vi "setSpeedByEnum.vi"(6 "Delay between send and receive [ms]":i32=1000, 8 "error in (no error)":errorcluster, 11 "CCD in":refnum<class "CCD.lvclass">) -> (0 "error out":errorcluster, 1 "ID":i32, 2 "results-JSON string":string, 3 "CCD out":refnum<class "CCD.lvclass">)   [LabVIEW 2023, in "CCD.lvclass"]
uses:
  CCD.lvclass
  CCD.lvclass/CCD.ctl
  SpeedTokenExampleEnum.ctl
panel:
  in  "speed":T1
  # "Connector Pane"
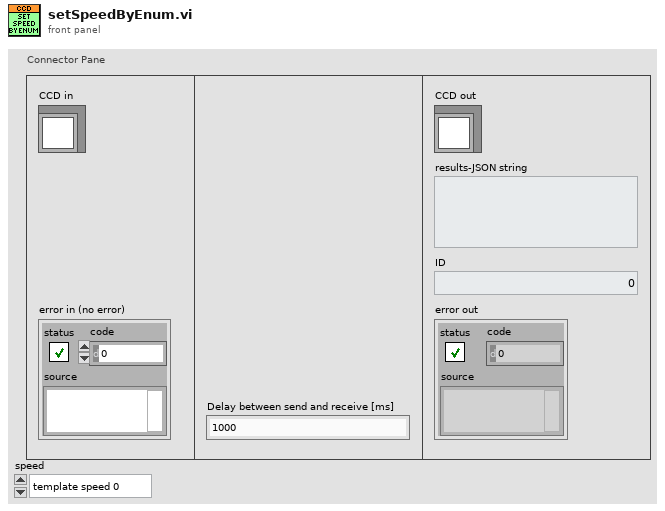
[diagram p1: front panel]
types:
  T1 = typedef "CCD.lvclass/SpeedTokenExampleEnum.ctl" = enum16{"template speed 0", "template speed 1", "template speed 2"}
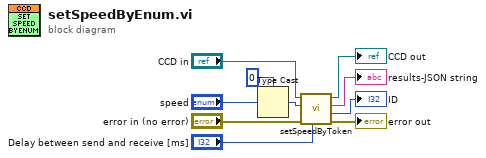
[diagram p0: block diagram]
diagram:
  n1 = Type Cast(type=u16 0, x="speed") -> (*(type *) &x=w2:u16)
  n2 = call "setSpeedByToken.vi"("Delay between send and receive [ms]"="Delay between send and receive [ms]", "error in (no error)"="error in (no error)", "speed token"=w2, "CCD in"="CCD in") -> ("error out"=→"error out":errorcluster, "ID"=→"ID":i32, "results-JSON string"=→"results-JSON string":string, "CCD out"=→"CCD out":refnum<class "CCD.lvclass">)  [unwired: 4 in]
